vi "random.vi"(6 "timeout (25000ms)":i32=25000, 8 "error in (no error)":errorcluster, 9 "max (100)":dbl=100.0, 10 "min (0)":dbl, 11 "daemon reference in":refnum<k5>) -> (0 "error out":errorcluster, 2 "random number":dbl, 3 "daemon reference out":refnum<k5>, 5 "command out":string="random")   [LabVIEW 2017]
doc: "<b>Command: </b>\"random\"\n\n<b>Description: </b> Instructs the Daemon to generate a random number (format DOUBLE).\n\n<b>Parameters: </b> \n\n 1. Min Value\n 2. Max Value\n____________________________________________\nDIPC 692 Daemon API 10.0.0.1\nSam Tee - Dyson Technology Ltd\nCopyright (c) 2024, Dyson Technology Ltd"
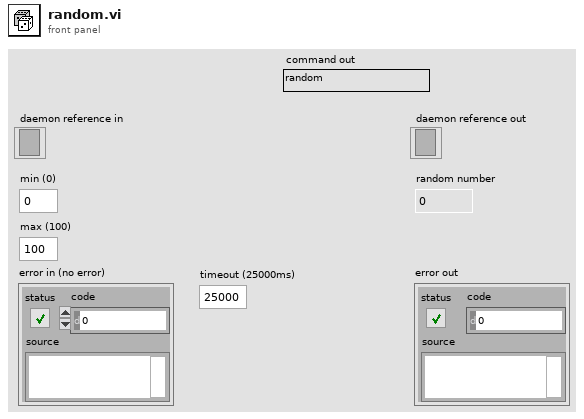
[diagram p1: front panel]
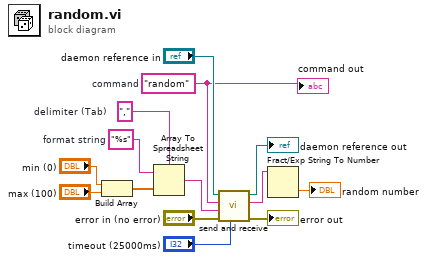
[diagram p0: block diagram]
diagram:
  w4 = ","  # delimiter (Tab)
  w5 = "%s"  # format string
  w12 = "random"  # command
  n1 = Build Array("min (0)", "max (100)") -> (w6:dbl[])
  n2 = Array To Spreadsheet String(delimiter (Tab)=w4, array=w6, 3:w5) -> (spreadsheet string=w3:string)
  n3 = call "send and receive.vi"("timeout (25000ms)"="timeout (25000ms)", "error in (no error)"="error in (no error)", "data"=w3, "command"=w12, "daemon reference in"="daemon reference in") -> ("error out"=→"error out":errorcluster, "response"=w2:string, "daemon reference out"=→"daemon reference out":refnum<k5>)  [unwired: 4 in]
  n4 = Fract/Exp String To Number(string=w2) -> (number=→"random number":dbl)  [unwired: 3 in, 1 out]
  "command out" <- w12
